vi "ClientProof.vi"(8 "error in (no error)":errorcluster, 9 "Authenticate Extra  Data":T1, 10 "Challenge data":T2, 11 "WampScramAuthenticator in":refnum<class "WampScramAuthenticator.lvclass">) -> (0 "error out":errorcluster, 2 "ClientProof":u8[](array[numeric]), 3 "WampScramAuthenticator out":refnum<class "WampScramAuthenticator.lvclass">)   [LabVIEW 2020, in "wamplv.lvlib" / "WampScramAuthenticator.lvclass"]
uses:
  WampScramAuthenticator.lvclass
  TypeDefs/Challenge data.ctl
  TypeDefs/Authenticate Extra data.ctl
  WampScramAuthenticator.lvclass/WampScramAuthenticator.ctl
  TypeDefs/HMAC parameters.ctl
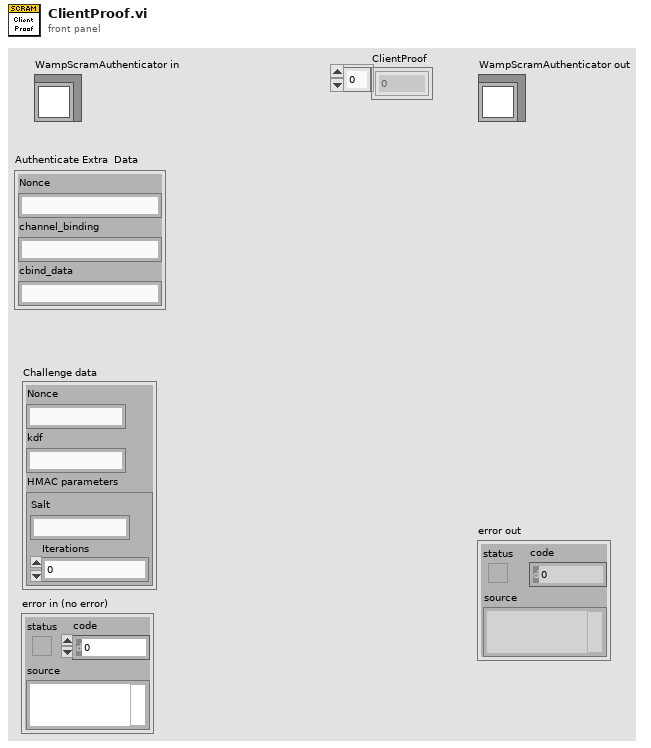
[diagram p1: front panel]
types:
  T1 = typedef "wamplv.lvlib/WampScramAuthenticator.lvclass/Authenticate Extra data.ctl" = cluster{"Nonce":string, "channel_binding":string, "cbind_data":string}
  T2 = typedef "wamplv.lvlib/WampScramAuthenticator.lvclass/Challenge data.ctl" = cluster{"Nonce":string, "kdf":string, "HMAC parameters":T3}
  T3 = typedef "wamplv.lvlib/WampScramAuthenticator.lvclass/HMAC parameters.ctl" = cluster{"Salt":string, "Iterations":i32}
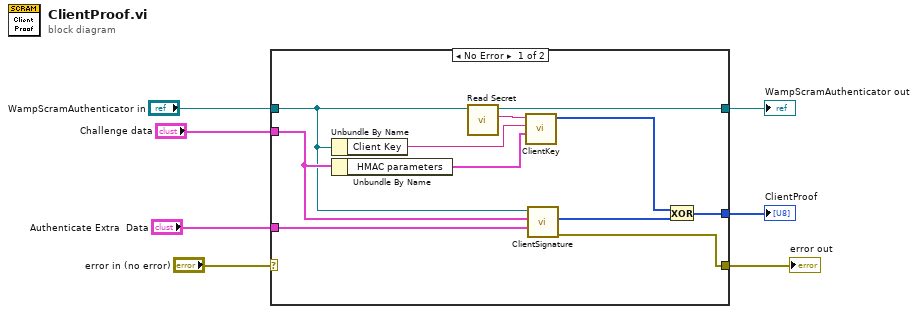
[diagram p0: block diagram]
diagram:
  n1 = case shown="No Error" "error in (no error)" {
    selector: "error in (no error)" -> [_ w20]
    tunnel: [w9 w20] -> w6
    tunnel: [w15 w19] -> w4
    tunnel: "WampScramAuthenticator in" -> [w8 w19]
    tunnel: "Challenge data" -> [w13 _]
    tunnel: "Authenticate Extra  Data" -> [w18 _]
    tunnel: [w16 _] -> w1
    frame No Error {
      n2 = Unbundle By Name(w8) -> ("Client Key"=w11:string)
      n3 = Unbundle By Name(w13) -> ("HMAC parameters"=w12:T3)
      n4 = call-dynamic "Read Secret.vi"("SecretBasedAuthenticatorBase in"=w8) -> ("Secret"=w14:string, "SecretBasedAuthenticatorBase out"=w15:refnum<class "WampScramAuthenticator.lvclass">)  [unwired: 8 in, 1 out]
      n5 = call "ClientKey.vi"("HMAC parameters"=w12, "Un-hashed client Key"=w11, "Secret"=w14) -> ("ClientKey"=w10:u8[])  [unwired: 8 in]
      n6 = call "ClientSignature.vi"("Authenticate Extra  Data"=w18, "Challenge data"=w13, "WampScramAuthenticator in"=w8) -> ("error out"=w9:errorcluster, "Client Signature"=w17:u8[])  [unwired: 6 in, 1 out]
      n7 = Exclusive Or(1:w17, 2:w10) -> (0:w16:u8[])
    }
    frame Error {
    }
  }
  "error out" <- w6
  "WampScramAuthenticator out" <- w4
  "ClientProof" <- w1
